vi "Frequency Response - Digital Mic.vi"() -> ()   [LabVIEW 2022 SP3]
uses:
  <vilib>/addons/_NISVFA/_Generation/Signal Generation/SV Signal/SV Signal.lvclass/SV Signal.ctl
  <vilib>/DAQmx/write.llb/DAQmx Write (Analog Wfm 1Chan NSamp).vi
  <vilib>/addons/_NISVFA/_Generation/Signal Generation/SV Signal/Write Leading Synchronization Pulse Enable.vi
  <vilib>/addons/_NISVFA/_Generation/Signal Generation/SV Signal/Read Total Samples.vi
  Program Files/NI/LVAddons/nisvt/1/examples/Sound and Vibration/Audio Measurements/subVIs/sv_Align Waveforms by Leading Sync Pulse.vi
  <vilib>/addons/_NISVFA/_Generation/Signal Generation/SV Signal/Read Synchronization Pulse Waveform.vi
  <vilib>/addons/_NISVFA/_Shared subVIs/Common/svc_Check for Waveform Parameter Continuity (N Ch).vi
  Program Files/NI/LVAddons/nisvt/1/examples/Sound and Vibration/Audio Measurements/subVIs/sv_Append Virtual Reference.vi
  <vilib>/addons/_NISVFA/_Shared subVIs/Common/svc_Get SV Channel Info.vi
  <vilib>/Analysis/baseanly.llb/Mean.vi
  <vilib>/Analysis/baseanly.llb/Mean (DBL).vi
  <vilib>/addons/_NISVFA/_Shared subVIs/Windowing/svfa_Scaled Time Domain Window (Array).vi
  <vilib>/addons/_NISVFA/_Generation/Signal Generation/SV Signal/Calculate Number of Remaining Samples.vi
  Program Files/NI/LVAddons/nisvt/1/examples/Sound and Vibration/Audio Measurements/subVIs/sv_Measure Delay for Active and Idle Channels.vi
  <vilib>/addons/_NISVFA/_Generation/Signal Generation/SV Signal/Read Leading Synchronization Pulse Enable.vi
  <vilib>/addons/_NISVFA/_Generation/Signal Generation/SV Signal/Read Trailing Synchronization Pulse Enable.vi
  <vilib>/addons/_NISVFA/_Shared subVIs/Common/svc_Check for Waveform Parameter Continuity (no state).vi
  <vilib>/addons/_NISVFA/_Shared subVIs/Common/sv_Get NI Property Name String.vi
  <vilib>/addons/_NISVFA/_Shared subVIs/Common/svc_Unit Label to Engineering Units.vi
  <vilib>/addons/_NISVFA/_Shared subVIs/Common/svc_Engineering Units to Unit Label.vi
  <vilib>/addons/_NISVFA/_Spectrum Processing/subVIs/svfa_Spectrum Info Window to windowTd Type Def.vi
  <vilib>/Analysis/4window.llb/Force Window.vi
  <vilib>/Analysis/4window.llb/Force Window (DBL).vi
  <vilib>/Analysis/4window.llb/Exponential Window.vi
  <vilib>/Analysis/4window.llb/Exponential Window (DBL).vi
  <vilib>/addons/Sound and Vibration/svt_Calibration/SV Measure Delay and Polarity and Coherence (Nx1).vi
  Program Files/NI/LVAddons/nisvt/1/examples/Sound and Vibration/Audio Measurements/subVIs/sv_Assign Delay to Idle Channels.vi
  <vilib>/addons/Sound and Vibration/svt_Calibration/SV Measure Delay and Polarity and Coherence.vi
  <vilib>/Analysis/_algsub.llb/Vector Norm.vi
  <vilib>/Analysis/_algsub.llb/Real Vector Norm.vi
  <vilib>/addons/_NISVFA/_Shared subVIs/Common/SV Get Data Subset.vi
  <vilib>/addons/_NISVFA/_Shared subVIs/Common/svc_Get Array Subset (Index).vi
  <vilib>/addons/_NISVFA/_Shared subVIs/Common/svc_Coerce Index and Length.vi
  <vilib>/addons/_NISVFA/_Shared subVIs/Common/svc_Conditional Merge Error.vi
  <vilib>/addons/_NISVFA/_Generation/Signal Generation/SV Discrete Sweep/SV Discrete Sweep.lvclass
  C:/Program Files/NI/LVAddons/nisvt/1/vi.lib/addons/_NISVFA/_Generation/Signal Generation/SV Signal/SV Signal.lvclass
  C:/Program Files/NI/LVAddons/nisvt/1/vi.lib/addons/_NISVFA/_Generation/Signal Generation/SV Function/SV Function.lvclass
  <vilib>/addons/_NISVFA/_Generation/Signal Generation/SV Discrete Sweep/Configure Frequency Sweep at Constant Amplitude.vi
  <vilib>/addons/_NISVFA/_Generation/Signal Generation/SV Signal/Write Ramp Parameters.vi
  <vilib>/addons/_NISVFA/_Generation/Signal Generation/SV Signal/Write Measurement Duration.vi
  <vilib>/addons/_NISVFA/_Generation/Signal Generation/SV Function/Write Measurement Cycles.vi
  <vilib>/addons/_NISVFA/_Generation/Signal Generation/SV Signal/Write Pre-Measurement Settling Duration.vi
  <vilib>/addons/_NISVFA/_Generation/Signal Generation/SV Function/Write Pre-Measurement Settling Cycles.vi
  <vilib>/addons/_NISVFA/_Generation/Signal Generation/SV Signal/Write Sample Rate.vi
  <vilib>/addons/_NISVFA/_Generation/Signal Generation/SV Signal/Read Generation State.vi
  <vilib>/addons/_NISVFA/_Generation/Signal Generation/SV Signal/Read System Timing Model.vi
  <vilib>/DAQmx/create/channels.llb/DAQmx Create Channel (AO-Voltage-Basic).vi
  <vilib>/DAQmx/configure/timing.llb/DAQmx Timing (Sample Clock).vi
  <vilib>/DAQmx/miscellaneous.llb/DAQmx Fill In Error Info.vi
  <vilib>/addons/_NISVFA/_Generation/Signal Generation/SV Signal/Write System Timing Model.vi
  <vilib>/addons/_NISVFA/_Shared subVIs/Data Objects/Waveforms (DBL)/SV Read Newest Data.vi
  <vilib>/measure/maresamp.llb/Resample Waveforms (single shot).vi
  <vilib>/measure/maresamp.llb/Resample Waveform (single shot).vi
  <vilib>/addons/_NISVFA/_Shared subVIs/Common/svc_Check dt for Equal Sample Rates.vi
  <vilib>/Waveform/TSOps.llb/Timestamp Subtract.vi
  <vilib>/Analysis/2dsp.llb/CrossCorrelation.vi
  <vilib>/Analysis/2dsp.llb/1D Cross Correlation (DBL).vi
  <vilib>/addons/_NISVFA/_Shared subVIs/Common/svc_Fit Quadratic to Max Three Points in Array.vi
  <vilib>/Utility/error.llb/Error Cluster From Error Code.vi
  <vilib>/addons/_NISVFA/_Shared subVIs/Common/svc_Caller VI Returned in Error Source.vi
  <vilib>/addons/_NISVFA/_Shared subVIs/Common/SV Remove Delays (1,N) from Waveforms (N Ch) (DBL).vi
  <vilib>/addons/_NISVFA/_Shared subVIs/Common/SV Remove Delays from Waveforms.vi
  <vilib>/addons/_NISVFA/_Generation/Signal Generation/SV Signal/Read Sample Rate.vi
  <vilib>/addons/_NISVFA/_Shared subVIs/Common/svc_Get Window Info.vi
  <vilib>/Analysis/0measdsp.llb/Scaled Time Domain Window.vi
  <vilib>/Analysis/0measdsp.llb/Scaled Time Domain Window (DBL).vi
  <vilib>/Analysis/baseanly.llb/Std Deviation and Variance.vi
  <vilib>/addons/_NISVFA/_Generation/Signal Generation/SV Signal/SV Signal.lvclass
  <vilib>/addons/_NISVFA/_Shared subVIs/Data Objects/Waveforms (DBL)/SV Read Next Measurement Data.vi
  <vilib>/addons/Sound and Vibration/svt_Level/SVL AC & DC Level (Time) (1 Ch).vi
  <vilib>/addons/_NISVFA/_Spectrum Processing/SVFA Extract Single Tone Information (Waveform) (1 Ch).vi
  <resource>/objmgr/daqmx.rc
  <vilib>/addons/_NISVFA/_Shared subVIs/Data Objects/Waveforms (DBL)/Waveforms (N Ch).lvclass
  Program Files/NI/LVAddons/nisvt/1/examples/Sound and Vibration/SoundVib_Audio Examples.lvlib
  C:/Program Files/NI/LVAddons/nisvt/1/vi.lib/addons/_NISVFA/_Generation/Signal Generation/SV Sinusoid/SV Sinusoid.lvclass
  C:/Program Files/NI/LVAddons/nisvt/1/vi.lib/addons/_NISVFA/_Generation/Signal Generation/SV Discrete Sweep/SV Discrete Sweep.lvclass
  <vilib>/DAQmx/configure/events/hardwareSignals.llb/DAQmx Export Signal (Most Signals).vi
  <vilib>/PDM Acquisition Toolkit/host/API/PDM Acquisition Toolkit.lvlib
  <vilib>/PDM Acquisition Toolkit/host/Classes/Tasks/PDM Tasks/Controls/Acquisition Mode.ctl
  <vilib>/PDM Acquisition Toolkit/host/Classes/Tasks/PDM Tasks/PDM Task.lvclass
  <vilib>/PDM Acquisition Toolkit/shared/controls/clock mode.ctl
  <vilib>/PDM Acquisition Toolkit/shared/PDM Shared.lvlib
  <vilib>/PDM Acquisition Toolkit/host/Classes/Session/Controls/FPGA Personality.ctl
  <vilib>/PDM Acquisition Toolkit/host/Classes/Session/DecoderSession.lvclass
  <vilib>/PDM Acquisition Toolkit/shared/controls/trigger polarity.ctl
  <vilib>/PDM Acquisition Toolkit/shared/controls/PXI trigger lines.ctl
  <vilib>/PDM Acquisition Toolkit/host/API/Controls/PDM Digital Start Trigger Cluster.ctl
  <vilib>/PDM Acquisition Toolkit/host/API/Public/Create Tasks/Create GPIO Output Task.vi
  <vilib>/PDM Acquisition Toolkit/host/API/Public/Create Tasks/Create PDM Input Task.vi
  <vilib>/PDM Acquisition Toolkit/host/API/Public/Configure/PDM Channel/Configure Microphone Sensitivity DBFS.vi
  <vilib>/PDM Acquisition Toolkit/host/API/Public/Configure/Triggering/Configure PDM Trigger (Digital Edge).vi
  <vilib>/PDM Acquisition Toolkit/host/API/Public/Configure/Timing/Configure Timing - PDM Input.vi
  <vilib>/PDM Acquisition Toolkit/host/API/Public/Read/Read PCM Waveform.vi
  <vilib>/PDM Acquisition Toolkit/host/API/Public/Clear/Clear PDM Input Task.vi
  <vilib>/PDM Acquisition Toolkit/host/Classes/Session/Controls/Logic Levels.ctl
  <vilib>/PDM Acquisition Toolkit/shared/controls/decimation order.ctl
panel:
  out "Actual PCM Clock Rate":dbl=47999.99987881165 format="%#_6p"
  out "Actual PDM Clock Rate":dbl=3071999.9922439456 format="%#_6p"
  in  "Microphone Sensitivity (dBFS)":dbl=-26.0 format="%#_13g"
  in  "PDM Clock Rate":dbl=3072000.0 format="%#_6p"
  in  "Decimation Factor":T1=64 items=["24"=24, "32"=32, "48"=48, "64"=64, "96"=96, "128"=128]
  in  "Logic Level":T2
  in  "Digital Output Channels":string="PXI1Slot5\\GPIO0"
  in  "PDM Channels":string="PXI1Slot5\\PDMi 0"
  in  "Tab Control":enum32{"Time Domain", "Frequency Response"}(tab)=enum."Frequency Response"
  out "Waveform Graph":waveform(dbl)[](graph)=[{"t0"=timestamp(3812131384.799704 s since 1904-01-01), "dt"=1.9531249997269942e-05, "Y"=array[65939 elements], "attributes"=variant("NI_ChannelName"=variant(string "PXI1Slot2/ai0"), "NI_UnitDescription"=variant(string "Pascals"), "NI_dBReference"=variant(dbl 2e-05))}]
  in  "sweep settings":T3(tab)=enum."EQ Settings"
  in  "speaker excitation channel":tag="PXI1Slot2/ao0"
  in  "number of steps":i32=50 min=1
  in  "amplitude":dbl=94.0 format="%.2p dBSPL"
  in  "frequency spacing":enum16{"Linear", "Logarithmic"}(ring)=enum."Logarithmic"
  in  "sweep range":cluster{"start":dbl, "stop":dbl}={"start"=10000.0, "stop"=300.0} {"stop" min=0.0 format="%.2f"; "start" min=0.0 format="%.2f"}
  in  "output voltage ratio":dbl=0.914 format="%#_g Pa/V"
  in  "EQ Action":T4(ring)=enum."Load and Apply EQ"
  in  "EQ File":path=path "C:/dev/digital-microphone/test/EQ_test.csv"
  in  "measurement":cluster{"time":dbl, "cycles":dbl}={"time"=0.001, "cycles"=25.0} {"cycles" min=5.0 max=1000.0 step=1.0; "time" min=0.0 max=5.0 step=0.0001 format="%.3f s"}
  in  "settling":cluster{"time":dbl, "cycles":dbl}={"time"=0.0, "cycles"=1.0} {"cycles" min=0.0 max=100.0 step=0.5; "time" min=0.0 max=5.0 step=0.0001 format="%.3f s"}
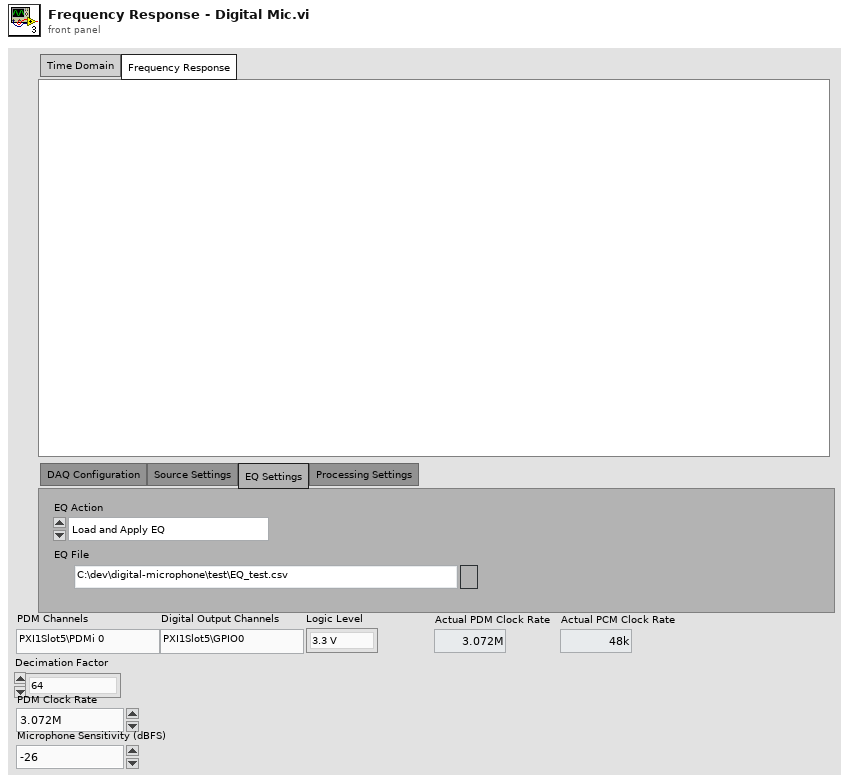
[diagram p1: front panel]
types:
  T1 = typedef "PDM Shared.lvlib/decimation order.ctl" = u16
  T2 = typedef "PDM Acquisition Class Library.lvlib/DecoderSession.lvclass/Logic Levels.ctl" = enum16{"3.3 V", "1.8 V", "1.2 V"}
  T3 = enum32{"DAQ Configuration", "Source Settings", "EQ Settings", "Processing Settings"}
  T4 = enum16{"Do Nothing", "Load and Apply EQ", "Save New EQ from Freq Response"}
  T5 = typedef "PDM Acquisition Toolkit.lvlib/PDM Digital Start Trigger Cluster.ctl" = cluster{"source":T6, "polarity":T7}
  T6 = typedef "PDM Shared.lvlib/PXI trigger lines.ctl" = enum16{"PXI_Trig0", "PXI_Trig1", "PXI_Trig2", "PXI_Trig3", "PXI_Trig4", "PXI_Trig5", "PXI_Trig6", "PXI_Trig7"}
  T7 = typedef "PDM Shared.lvlib/trigger polarity.ctl" = enum16{"Rising Edge", "Falling Edge"}
  T8 = typedef "PDM Acquisition Class Library.lvlib/DecoderSession.lvclass/FPGA Personality.ctl" = enum16{"PDM acquisition", "PDM generation", "I2S acquisition", "I2S generation", "PCM flexible", "PCM acquisition", "PCM generation"}
  T9 = typedef "PDM Shared.lvlib/clock mode.ctl" = enum16{"divided clock", "DDS"}
  T10 = typedef "PDM Acquisition Class Library.lvlib/PDM Task.lvclass/Acquisition Mode.ctl" = enum16{"Finite", "Continuous"}
  T11 = cluster{"profile":enum16{"Linear", "Half cosine"}, "durations [s]":cluster{"ramp-up":dbl, "transition":dbl, "ramp-down":dbl}}
  T12 = cluster{"frequency [Hz]":dbl, "amplitude [EU pk]":dbl, "phase (deg)":dbl}
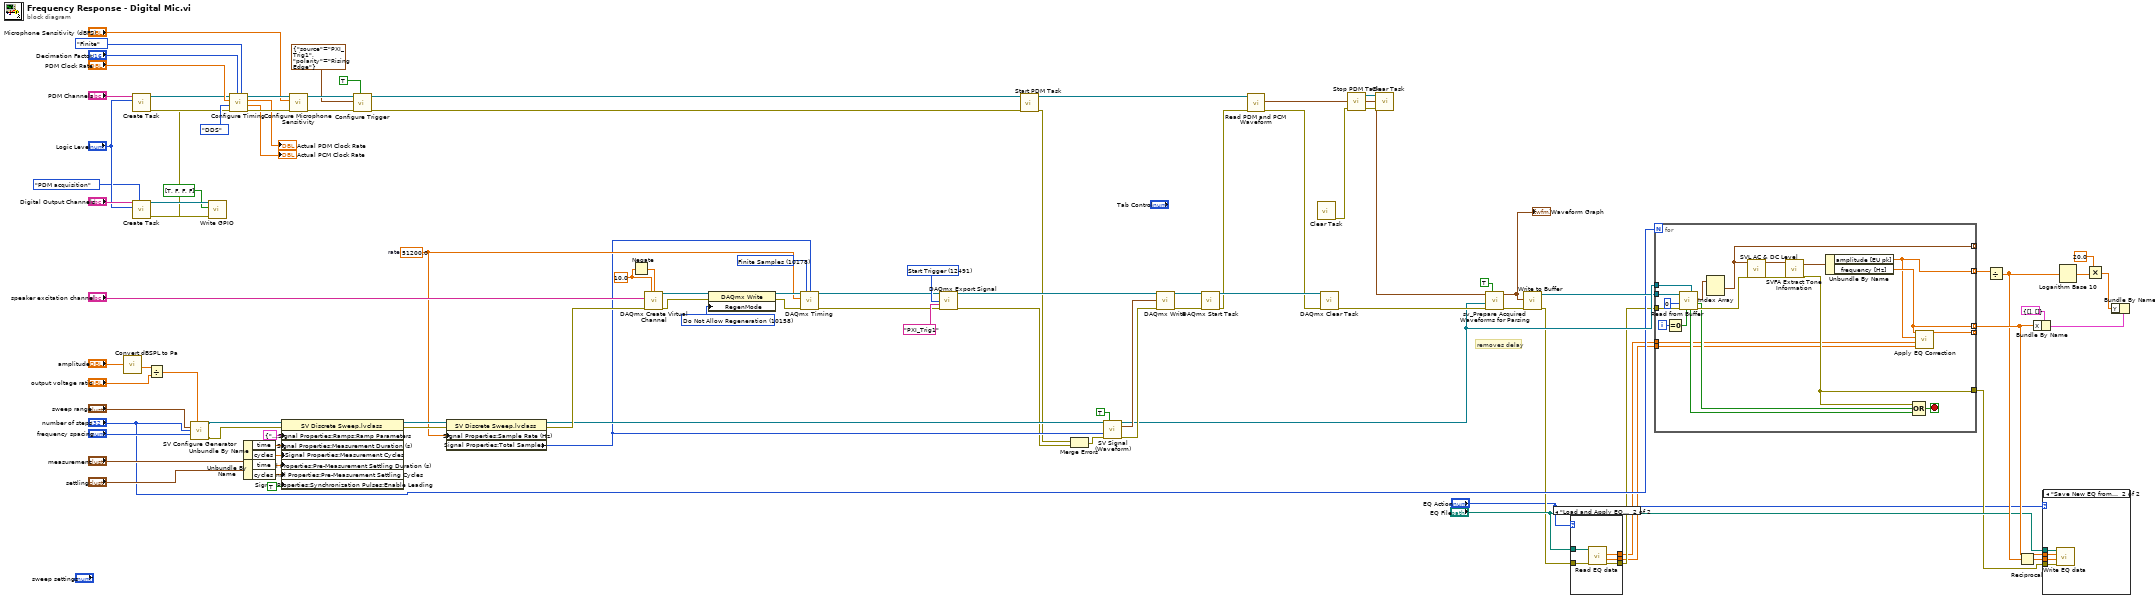
[diagram p0: block diagram]
diagram:
  w42 = 12491 items=["AI Convert Clock"=12484, "10MHz Reference Clock"=12536, "20MHz Timebase Clock"=12486, "Sample Clock"=12487, "Advance Trigger"=12488, "Reference Trigger"=12490, "Start Trigger"=12491, "Advance Complete Event"=12492, "AI Hold Complete Event"=12493, "Counter Output Event"=12494, "Change Detection Event"=12511, "Watchdog Timer Expired Event"=12512] ("signal")
  w86 = 10158 items=["Allow Regeneration"=10097, "Do Not Allow Regeneration"=10158] ("RegenMode")
  w88 = 10.0 ("maximum value")
  w89 = 10178 items=["Finite Samples"=10178, "Continuous Samples"=10123, "Hardware Timed Single Point"=12522] ("sample mode")
  w76 = 51200.0  # rate
  # "removes delay"
  n1 = call "Convert dBSPL to Pa.vi"("dB SPL"="amplitude") -> ("Pa pk"=w45:dbl)  [unwired: 9 in, 1 out]
  n2 = call-poly <vilib>:"Create Task.vi"("FPGA personality"=FPGA_Personality."PDM acquisition", "logic level"="Logic Level", "channel list"="Digital Output Channels") -> ("error out"=w24:errorcluster, "GPIO output task out"=w25:refnum<data-value>)  [unwired: 7 in]
  n3 = Divide(x=w45, y="output voltage ratio") -> (x/y=w90:dbl)
  n4 = call-poly <vilib>:"SV Configure Generator.vi"("amplitude"=w90, "frequency range [Hz]"="sweep range", "number of steps"="number of steps", "profile"="frequency spacing") -> ("signal configuration"=w98:refnum<class "SV Discrete Sweep.lvclass">, "error out"=w97:errorcluster)  [unwired: 10 in]
  n5 = call <vilib>:"Write GPIO.vi"("error in"=w24, "data"=bool[] [TRUE, FALSE, FALSE, FALSE] ("Output Values"), "GPIO output task in"=w25) -> ("error out"=w8:errorcluster, "GPIO output task out"=w27:refnum<data-value>)  [unwired: 7 in]
  n6 = call-poly <vilib>:"Create Task.vi"("error in"=w8, "logic level"="Logic Level", "channel list"="PDM Channels") -> ("error out"=w22:errorcluster, "PDM input task out"=w23:refnum<data-value>)  [unwired: 7 in]
  n7 = call-poly <vilib>:"Configure Timing.vi"("acquisition mode"=Acquisition_Mode."Finite" ("Acquisition Mode"), "decimation factor"="Decimation Factor", "error in"=w22, "clock mode"=clock_mode."DDS" ("Clock Type"), "PDM clock rate"="PDM Clock Rate", "PDM input task in"=w23) -> ("error out"=w28:errorcluster, "actual PCM clock rate"=→"Actual PCM Clock Rate":dbl, "actual PDM clock rate"=→"Actual PDM Clock Rate":dbl, "PDM input task out"=w29:refnum<data-value>, "number of PCM samples"=w16:i32)  [unwired: 1 in]
  n8 = Unbundle By Name("measurement") -> ("time"=w100:dbl, "cycles"=w99:dbl)
  n9 = Unbundle By Name("settling") -> ("time"=w102:dbl, "cycles"=w101:dbl)
  n10 = property class="SV Discrete Sweep.lvclass"(reference=w98, error in=w97, "Signal Properties:Ramps:Ramp Parameters"=T11 {"profile"=enum."Half cosine", "durations [s]"={"ramp-up"=0.01, "transition"=0.0, "ramp-down"=0.01}} ("Ramp Parameters"), "Signal Properties:Measurement Duration (s)"=w100, "Signal Properties:Measurement Cycles"=w99, "Signal Properties:Pre-Measurement Settling Duration (s)"=w102, "Signal Properties:Pre-Measurement Settling Cycles"=w101, "Signal Properties:Synchronization Pulses:Enable Leading"=TRUE ("Synchronization Pulses:Enable Leading")) -> (reference out=w78:refnum<class "SV Discrete Sweep.lvclass">, error out=w79:errorcluster)
  n11 = call-poly <vilib>:"Configure Microphone Sensitivity.vi"("error in"=w28, "microphone sensitivity (dBFS)"="Microphone Sensitivity (dBFS)", "PDM input task in"=w29) -> ("error out"=w12:errorcluster, "PDM input task out"=w15:refnum<data-value>)  [unwired: 7 in]
  n12 = call-poly <vilib>:"Configure Trigger.vi"("remove filter delay samples"=TRUE, "error in"=w12, "trigger configuration"=T5 {"source"=enum."PXI_Trig1", "polarity"=enum."Rising Edge"}, "PDM input task in"=w15) -> ("error out"=w13:errorcluster, "PDM input task out"=w14:refnum<data-value>)  [unwired: 6 in]
  n13 = property on="Property Node" class="SV Discrete Sweep.lvclass"(reference=w78, error in=w79, "Signal Properties:Sample Rate (Hz)"=w76) -> (reference out=w74:refnum<class "SV Discrete Sweep.lvclass">, error out=w77:errorcluster, "Signal Properties:Total Samples"=w73:i32)
  n14 = Negate(x=w88) -> (-x=w87:dbl)
  n15 = call-poly <vilib>:"DAQmx Create Virtual Channel.vi"("maximum value"=w88, "minimum value"=w87, "physical channels"="speaker excitation channel", "error in"=w77) -> ("task out"=w85:refnum<k21>, "error out"=w83:errorcluster)  [unwired: 10 in]
  n16 = property class="DAQmx Write"(reference=w85, error in=w83, "RegenMode"=w86) -> (reference out=w84:refnum<k21>, error out=w82:errorcluster)
  n17 = call-poly <vilib>:"DAQmx Timing.vi"("task/channels in"=w84, "sample mode"=w89, "samples per channel"=w73, "rate"=w76, "error in"=w82) -> ("task out"=w38:refnum<k21>, "error out"=w37:errorcluster)  [unwired: 9 in]
  n18 = call-poly <vilib>:"DAQmx Export Signal.vi"("task/channels in"=w38, "signal"=w42, "output terminal"="PXI_Trig1", "error in"=w37) -> ("task out"=w40:refnum<k21>, "error out"=w39:errorcluster)  [unwired: 10 in]
  n19 = call <vilib>:"Start PDM Task.vi"("error in"=w13, "PDM input task in"=w14) -> ("error out"=w7:errorcluster, "PDM input task out"=w33:refnum<data-value>)  [unwired: 8 in]
  n20 = Merge Errors(w7, w39) -> (w72:errorcluster)
  n21 = call-dynamic "SV Signal (Waveform).vi"("signal configuration"=w74, "reset"=TRUE, "samples"=w73, "error in (no error)"=w72) -> ("signal configuration"=w63:refnum<class "SV Discrete Sweep.lvclass">, "output waveform"=w70:waveform(dbl), "error out"=w71:errorcluster)  [unwired: 6 in, 3 out]
  n22 = call-poly <vilib>:"DAQmx Write.vi"("task/channels in"=w40, "data"=w70, "error in"=w71) -> ("task out"=w68:refnum<k21>, "error out"=w69:errorcluster)  [unwired: 10 in, 1 out]
  n23 = call <vilib>:"DAQmx Start Task.vi"("task/channels in"=w68, "error in"=w69) -> ("task out"=w67:refnum<k21>, "error out"=w5:errorcluster)  [unwired: 12 in]
  n24 = call-poly <vilib>:"Read PDM and PCM Waveform.vi"("error in"=w5, "PDM input task in"=w33) -> ("error out"=w4:errorcluster, "PCM waveforms"=w6:waveform(dbl)[], "samples per channel"=w17:i32)  [unwired: 5 in, 2 out]
  n25 = call-poly <vilib>:"Clear Task.vi"() -> ("error out"=w1:errorcluster)  [unwired: 11 in]
  n26 = call <vilib>:"DAQmx Clear Task.vi"("task in"=w67, "error in"=w4) -> ("error out"=w65:errorcluster)  [unwired: 13 in]
  n27 = call <vilib>:"Stop PDM Task.vi"("error in"=w1) -> ("error out"=w2:errorcluster, "PDM input task out"=w3:refnum<data-value>)  [unwired: 9 in]
  n28 = call-poly <vilib>:"Clear Task.vi"("error in"=w2, "PDM input task in"=w3) -> ()  [unwired: 9 in, 1 out]
  n29 = call "sv_Prepare Acquired Waveforms for Parsing.vi"("restart (F)"=TRUE, "error in"=w65, "SV Signal"=w63, "acquired channel waveforms"=w6) -> ("error out"=w64:errorcluster, "aligned channel waveforms"=w55:waveform(dbl)[])  [unwired: 5 in, 1 out]
  "Waveform Graph" <- w55
  n30 = call <vilib>:"Write to Buffer.vi"("error in (no error)"=w64, "waveforms"=w55) -> ("error out"=w50:errorcluster, "buffer out"=w62:refnum<data-value>)  [unwired: 7 in, 1 out]
  n31 = case shown="\"Load and Apply EQ\"" "EQ Action" {
    tunnel: "EQ File" -> [_ w109]
    tunnel: w50 -> [w104 w108]
    tunnel: [w104 w107] -> w49
    tunnel: [_ w106] -> w48
    tunnel: [_ w105] -> w47
    frame "Do Nothing", Default {
    }
    frame "Load and Apply EQ" {
      n32 = call "Read EQ data.vi"("error in (no error)"=w108, "file path"=w109) -> ("error out"=w107:errorcluster, "gain correction (x/y)"=w105:dbl[], "frequency"=w106:dbl[])  [unwired: 7 in]
    }
  }
  n33 = for {
    N: "number of steps" -> [_]
    tunnel: w62 -> [w127]
    tunnel: w63 -> [w126]
    tunnel: w49 -> [w125]
    tunnel: [w114] -> w54 mode=indexing
    tunnel: [w121] -> _ mode=indexing
    tunnel: [w113] -> w59 mode=indexing
    tunnel: w48 -> [w112]
    tunnel: w47 -> [w111]
    tunnel: [w115] -> w46
    tunnel: [w110] -> _ mode=indexing
    i -> [w120]
    stop <- w122 stop-if-true
    n34 = Equal To 0?(x=w120) -> (x = 0?=w119:bool)
    n35 = call-poly <vilib>:"Read from Buffer.vi"("test signal configuration"=w126, "reset start (F)"=w119, "error in (no error)"=w125, "timeout (1000 ms)"=0, "buffer"=w127) -> ("error out"=w130:errorcluster, "end of buffer"=w123:bool, "waveforms subset"=w124:waveform(dbl)[], "done"=w129:bool)  [unwired: 2 in, 1 out]
    n36 = Index Array(array=w124) -> (element #1=w121:waveform(dbl))  [unwired: 2 in, 1 out]
    n37 = call-poly <vilib>:"SVL AC & DC Level.vi"("scaled signal [EU]"=w121, "error in (no error)"=w130) -> ("AC signal [EU]"=w118:waveform(dbl), "error out"=w117:errorcluster)  [unwired: 12 in, 4 out]
    n38 = call-poly <vilib>:"SVFA Extract Tone Information.vi"("scaled signal [EU]"=w118, "error in"=w117) -> ("detected tone"=w116:T12, "error out"=w115:errorcluster)  [unwired: 15 in, 1 out]
    n39 = Unbundle By Name(w116) -> ("amplitude [EU pk]"=w113:dbl, "frequency [Hz]"=w114:dbl)
    n40 = Compound Arithmetic op=OR(w115, w123, w129) -> (w122:bool)
    n41 = call "Apply EQ Correction.vi"("gain correction (x/y)"=w111, 9:"frequency"=w112, "amplitude"=w113, 11:"frequency"=w114) -> ("corrected amplitude"=w110:dbl)  [unwired: 7 in]
  }
  n42 = Divide(x=w59) -> (x/y=w53:dbl[])  [unwired: 1 in]
  n43 = Reciprocal(x=w53) -> (1/x=w52:dbl[])
  n44 = Bundle By Name(cluster=cluster{"X":dbl[], "Y":dbl[]} {"X"=[], "Y"=[]} ("THD vs Amplitude"), "X"=w54) -> (w44:cluster{"X":dbl[], "Y":dbl[]})
  n45 = case shown="\"Save New EQ from Freq Response\"" "EQ Action" {
    tunnel: w54 -> [_ w134]
    tunnel: w52 -> [_ w133]
    tunnel: "EQ File" -> [_ w132]
    tunnel: w46 -> [_ w131]
    frame "Do Nothing", Default {
    }
    frame "Save New EQ from Freq Response" {
      n46 = call "Write EQ data.vi"("error in (no error)"=w131, "gain correction (x/y)"=w133, "frequency"=w134, "file path"=w132) -> ()  [unwired: 7 in, 1 out]
    }
  }
  n47 = Logarithm Base 10(1:w53) -> (0:w58:dbl[])
  n48 = Multiply(x=20.0, y=w58) -> (x*y=w57:dbl[])
  n49 = Bundle By Name(cluster=w44, "Y"=w57) -> ()  [unwired: 1 out]
